vi "Proceed.vi"(7 "component is ready (Y)":bool=TRUE, 8 "error in (no error)":errorcluster, 10 "ProceedMessage":refnum<class "ProceedMessage.lvclass">=refnum, 11 "PockelCell in":refnum<class "PockelCell.lvclass">) -> (0 "error out":errorcluster, 3 "PockelCell out":refnum<class "PockelCell.lvclass">)   [LabVIEW 2012, in "PockelCell.lvclass"]
uses:
  PockelCell.lvclass
  <vilib>/Distrio/Murmex/Murmex/Murmex.lvclass
  Murmex/LabVIEW/Murmex/ProceedMessage/ProceedMessage.lvclass
panel:
  # "This method is called when the PROCEED\ntrigger is sent. \n\nOverride this method when your component needs to\nrespond to this trigger. \n\nCall parent for proper implementation"
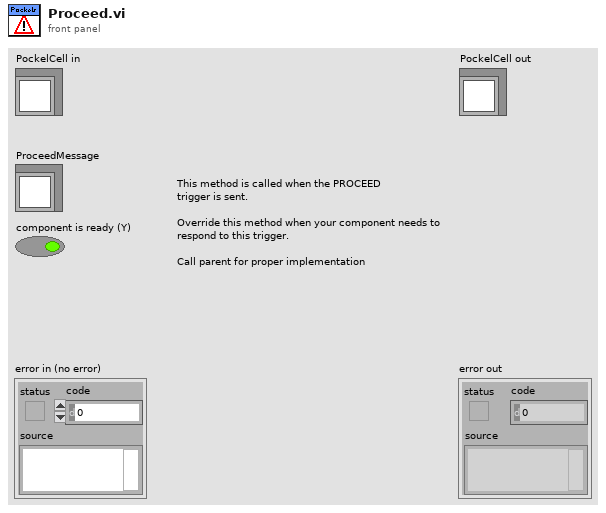
[diagram p1: front panel]
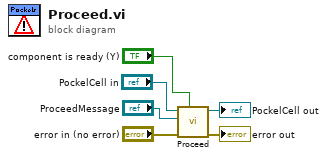
[diagram p0: block diagram]
diagram:
  n1 = call-parent "Proceed.vi"("component is ready (Y)"="component is ready (Y)", "error in (no error)"="error in (no error)", "ProceedMessage"="ProceedMessage", "Murmex in"="PockelCell in") -> ("error out"=→"error out":errorcluster, "Murmex out"=→"PockelCell out":refnum<class "PockelCell.lvclass">)  [unwired: 6 in]
